vi "check_generate_new_tap_array.vi"(0 "Input References Cluster":T2, 1 "Input values cluster":T1={"Value"=FALSE, "Value"=-1000.0, "Value"=-1000.0, "Value"=1000, "Value"=1000}) -> (2 "Output References Cluster":T2, 3 "Need new tap array?":bool, 4 "Output Values Cluster":T1={"Value"=FALSE, "Value"=-1000.0, "Value"=-1000.0, "Value"=1000, "Value"=1000})   [LabVIEW 2010]
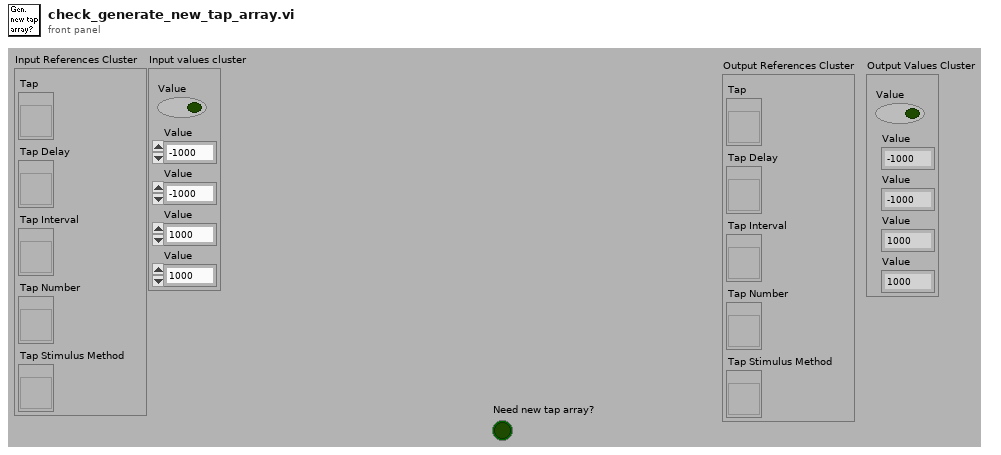
[diagram p1: front panel]
types:
  T1 = cluster{"Value":bool, "Value":dbl, "Value":dbl, "Value":i32, "Value":u16}
  T2 = cluster{"Tap":refnum<vi>, "Tap Delay":refnum<vi>, "Tap Interval":refnum<vi>, "Tap Number":refnum<vi>, "Tap Stimulus Method":refnum<vi>}
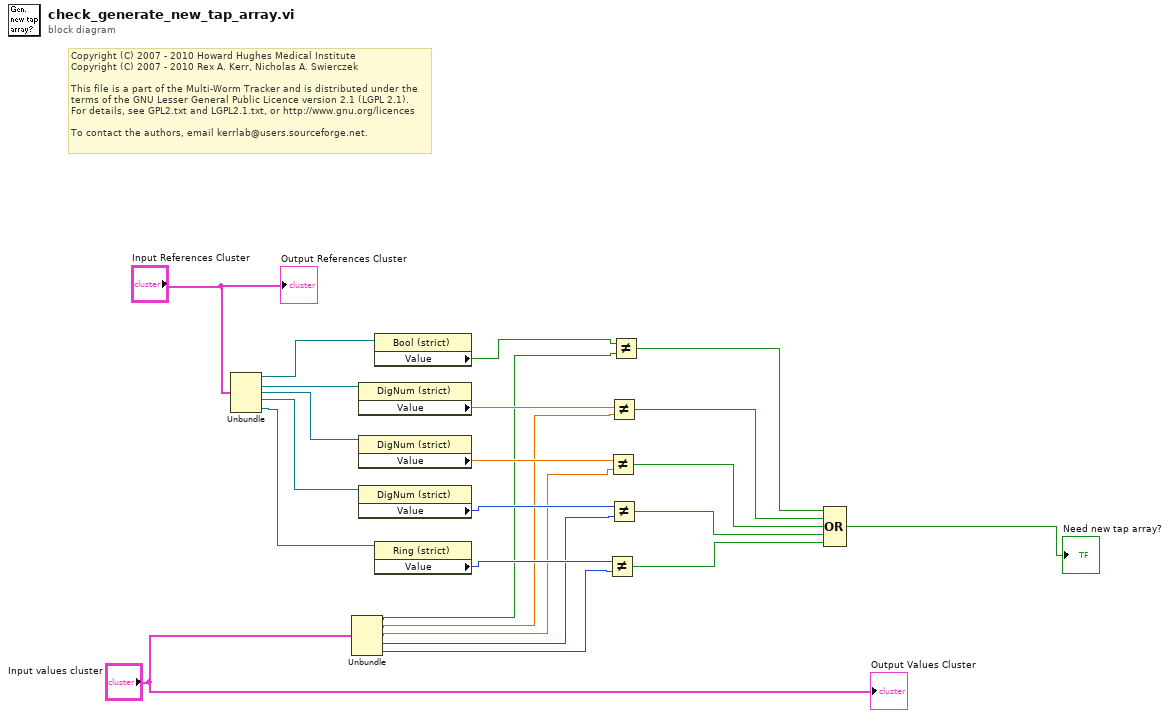
[diagram p0: block diagram]
diagram:
  # "Copyright (C) 2007 - 2010 Howard Hughes Medical Institute\nCopyright (C) 2007 - 2010 Rex A. Kerr, Nicholas A. Swierczek\n \nThis file is a part of the Multi-Worm Tracker and is distributed under the\nterms of the GNU Lesser General Public Licence version 2.1 (LGPL 2.1).\nFor details, see GPL2.txt and LGPL2.1.txt, or http://www.gnu.org/licences\n \nTo contact the authors, email kerrlab@users.sourceforge.net."
  n1 = Unbundle("Input References Cluster") -> ("Tap"=w22:refnum<vi>, "Tap Delay"=w21:refnum<vi>, "Tap Interval"=w20:refnum<vi>, "Tap Number"=w19:refnum<vi>, "Tap Stimulus Method"=w18:refnum<vi>)
  n2 = Unbundle("Input values cluster") -> ("Value"=w11:bool, "Value"=w10:dbl, "Value"=w9:dbl, "Value"=w8:i32, "Value"=w7:u16)
  n3 = property class="DigNum (strict)"(reference=w21) -> ("Value"=w16:dbl)  [unwired: 1 in, 2 out]
  n4 = property class="DigNum (strict)"(reference=w20) -> ("Value"=w15:dbl)  [unwired: 1 in, 2 out]
  n5 = property class="DigNum (strict)"(reference=w19) -> ("Value"=w14:i32)  [unwired: 1 in, 2 out]
  n6 = property class="Bool (strict)"(reference=w22) -> ("Value"=w17:bool)  [unwired: 1 in, 2 out]
  n7 = property class="Ring (strict)"(reference=w18) -> ("Value"=w13:u16)  [unwired: 1 in, 2 out]
  n8 = Not Equal?(x=w13, y=w7) -> (x != y?=w2:bool)
  n9 = Not Equal?(x=w15, y=w9) -> (x != y?=w4:bool)
  n10 = Not Equal?(x=w16, y=w10) -> (x != y?=w5:bool)
  n11 = Not Equal?(x=w14, y=w8) -> (x != y?=w3:bool)
  n12 = Not Equal?(x=w17, y=w11) -> (x != y?=w6:bool)
  n13 = Compound Arithmetic op=OR(w6, w5, w4, w3, w2) -> (→"Need new tap array?":bool)
  "Output References Cluster" <- "Input References Cluster"
  "Output Values Cluster" <- "Input values cluster"
